vi "SetOutputDelay.vi"(0 "VISA resource name":refnum<visa-resource-name>, 1 "Skew (s)":dbl, 2 "Selection":u8(ring) items=["Value", "Minimum", "Maximum", "Default"], 3 "error in (no error)":errorcluster, 4 "Channel (0: Channel 1)":u16(ring) items=["Channel 1", "Channel 2", "Channel 3", "Channel 4", "Channel 5", "Channel 6", "Channel 7", "Channel 8"]) -> (5 "VISA resource name out":refnum<visa-resource-name>, 6 "error out":errorcluster)   [LabVIEW 2020, in "Active Technologies AWG3000.lvlib"]
uses:
  Active Technologies AWG3000.lvlib
panel:
  out "VISA STRING":string
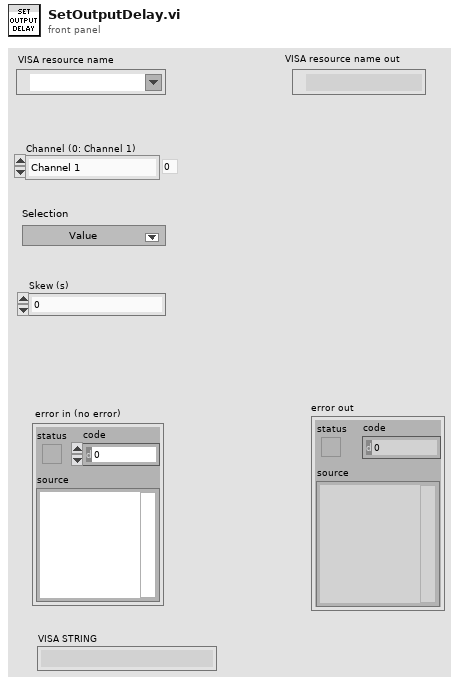
[diagram p1: front panel]
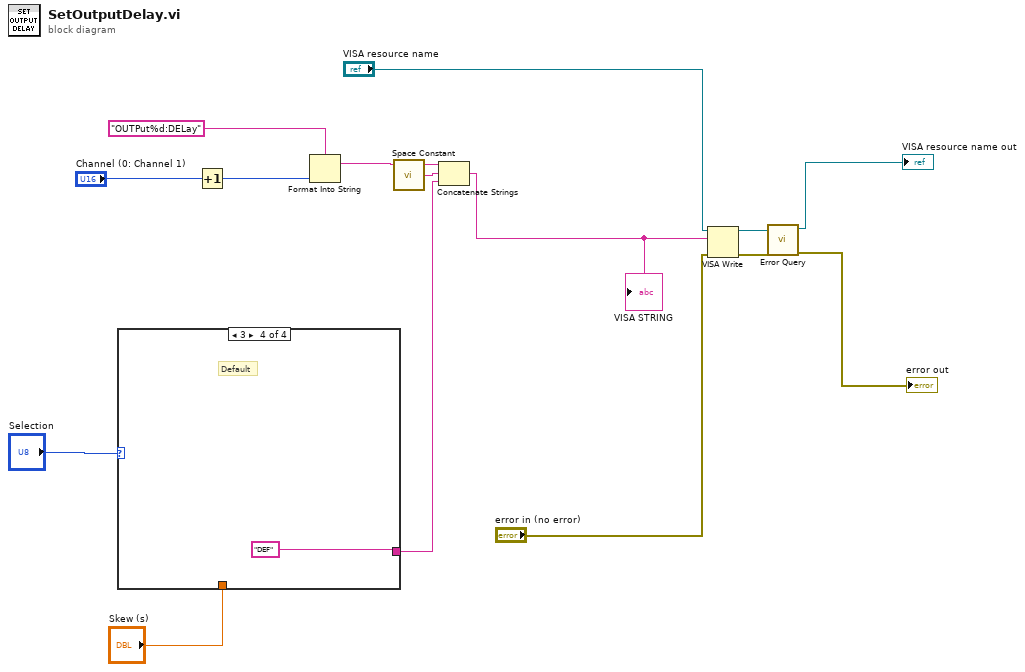
[diagram p0: block diagram]
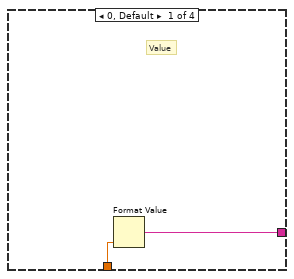
[diagram p2: hidden frame]
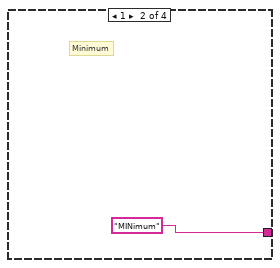
[diagram p3: hidden frame]
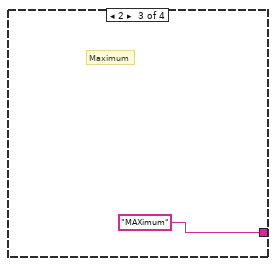
[diagram p4: hidden frame]
diagram:
  n1 = case shown="3" "Selection" {
    tunnel: "Skew (s)" -> [w17 _ _ _]
    tunnel: [w16 "MINimum" "MAXimum" "DEF"] -> w3
    frame 0, Default {
      # "Value"
      n2 = Format Value(value (0)=w17) -> (output string=w16:string)  [unwired: 2 in]
    }
    frame 1 {
      # "Minimum"
    }
    frame 2 {
      # "Maximum"
    }
    frame 3 {
      # "Default"
    }
  }
  n3 = Increment(x="Channel (0: Channel 1)") -> (x+1=w7:u16)
  n4 = Format Into String(format string="OUTPut%d:DELay" ("write buffer"), w7) -> (resulting string=w6:string)  [unwired: 2 in, 1 out]
  n5 = call <vilib>:"Space Constant.vi"() -> ("String"=w5:string)
  n6 = Concatenate Strings(w6, w5, w3) -> (w2:string)
  "VISA STRING" <- w2
  n7 = VISA Write(VISA resource name="VISA resource name", write buffer=w2, error in (no error)="error in (no error)") -> (VISA resource name out=w13:refnum<visa-resource-name>, error out=w12:errorcluster)  [unwired: 1 out]
  n8 = call "Error Query.vi"("error in (no error)"=w12, "VISA resource name"=w13) -> ("error out"=→"error out":errorcluster, "VISA resource name out"=→"VISA resource name out":refnum<visa-resource-name>)  [unwired: 6 in, 2 out]
